vi "MSGR Send (Refnum).vi"(0 "Msg":string, 1 "MSGR Q":refnum<queue>, 5 "Parameters":string, 7 "Reply?":bool, 9 "ReplyQ":string, 11 "error in (no error)":errorcluster, 12 "timeout in ms (-1)":i32=-1) -> (8 "timed out?":bool, 15 "error out":errorcluster)   [LabVIEW 2018]
uses:
  MSGR Q Data TypeDef.ctl
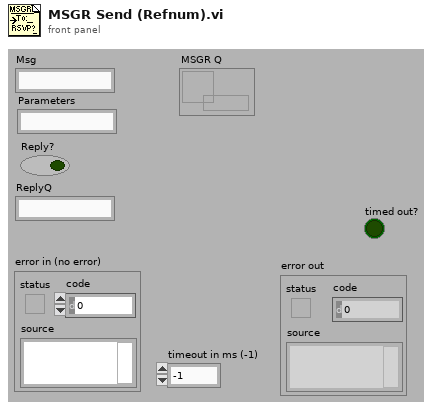
[diagram p1: front panel]
types:
  T1 = typedef "MSGR Q Data TypeDef.ctl" = cluster{"Msg":string, "Parameters":string, "Reply?":bool, "ReplyQ":string}
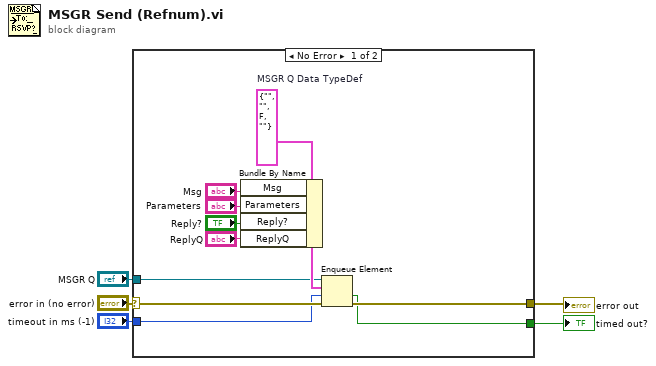
[diagram p0: block diagram]
diagram:
  n1 = case shown="No Error" "error in (no error)" {
    selector: "error in (no error)" -> [w8 w17]
    tunnel: [w12 w17] -> w5
    tunnel: "MSGR Q" -> [w9 _]
    tunnel: "timeout in ms (-1)" -> [w7 _]
    tunnel: [w6 _] -> w1
    frame No Error {
      w11 = T1 {"Msg"="", "Parameters"="", "Reply?"=FALSE, "ReplyQ"=""}  # MSGR Q Data TypeDef
      n2 = Bundle By Name(cluster=w11, "Msg"="Msg", "Parameters"="Parameters", "Reply?"="Reply?", "ReplyQ"="ReplyQ") -> (w16:T1)
      n3 = Enqueue Element(queue=w9, element=w16, timeout in ms (-1)=w7, error in (no error)=w8) -> (timed out?=w6:bool, error out=w12:errorcluster)  [unwired: 1 out]
    }
    frame Error {
    }
  }
  "error out" <- w5
  "timed out?" <- w1
